vi "Error Tree Value Change and Cycle Numbers.vi"(8 "error in (no error)":errorcluster, 11 "Error Log in":refnum<class "Error Log.lvclass">) -> (0 "error out":errorcluster, 3 "Error Log out":refnum<class "Error Log.lvclass">)   [LabVIEW 2023, in "Data Analysis.lvlib" / "Error Log.lvlib" / "Error Log.lvclass"]
uses:
  Error Log.lvclass
  Error Log.lvclass/Error Log.ctl
  HardwareAbstractionLayer_LVOOP/Database/Database.lvclass
  Data Analysis.lvlib
  <vilib>/Utility/miscctls.llb/LVRowAndColumnUnsignedTypeDef.ctl
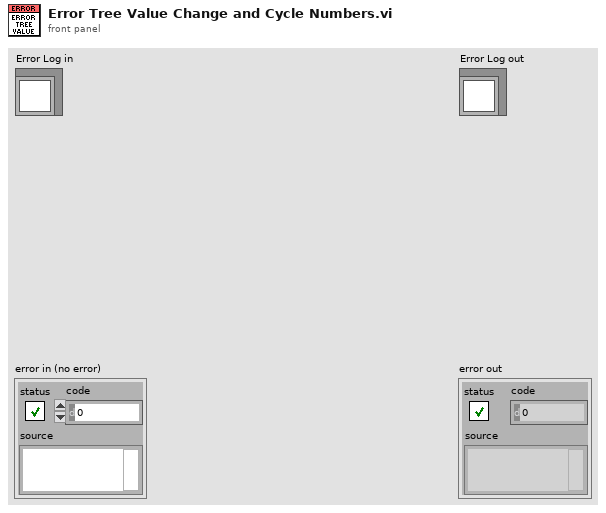
[diagram p1: front panel]
types:
  T1 = typedef "LVRowAndColumnUnsignedTypeDef.ctl" = cluster{"Row":u32, "Column":u32}
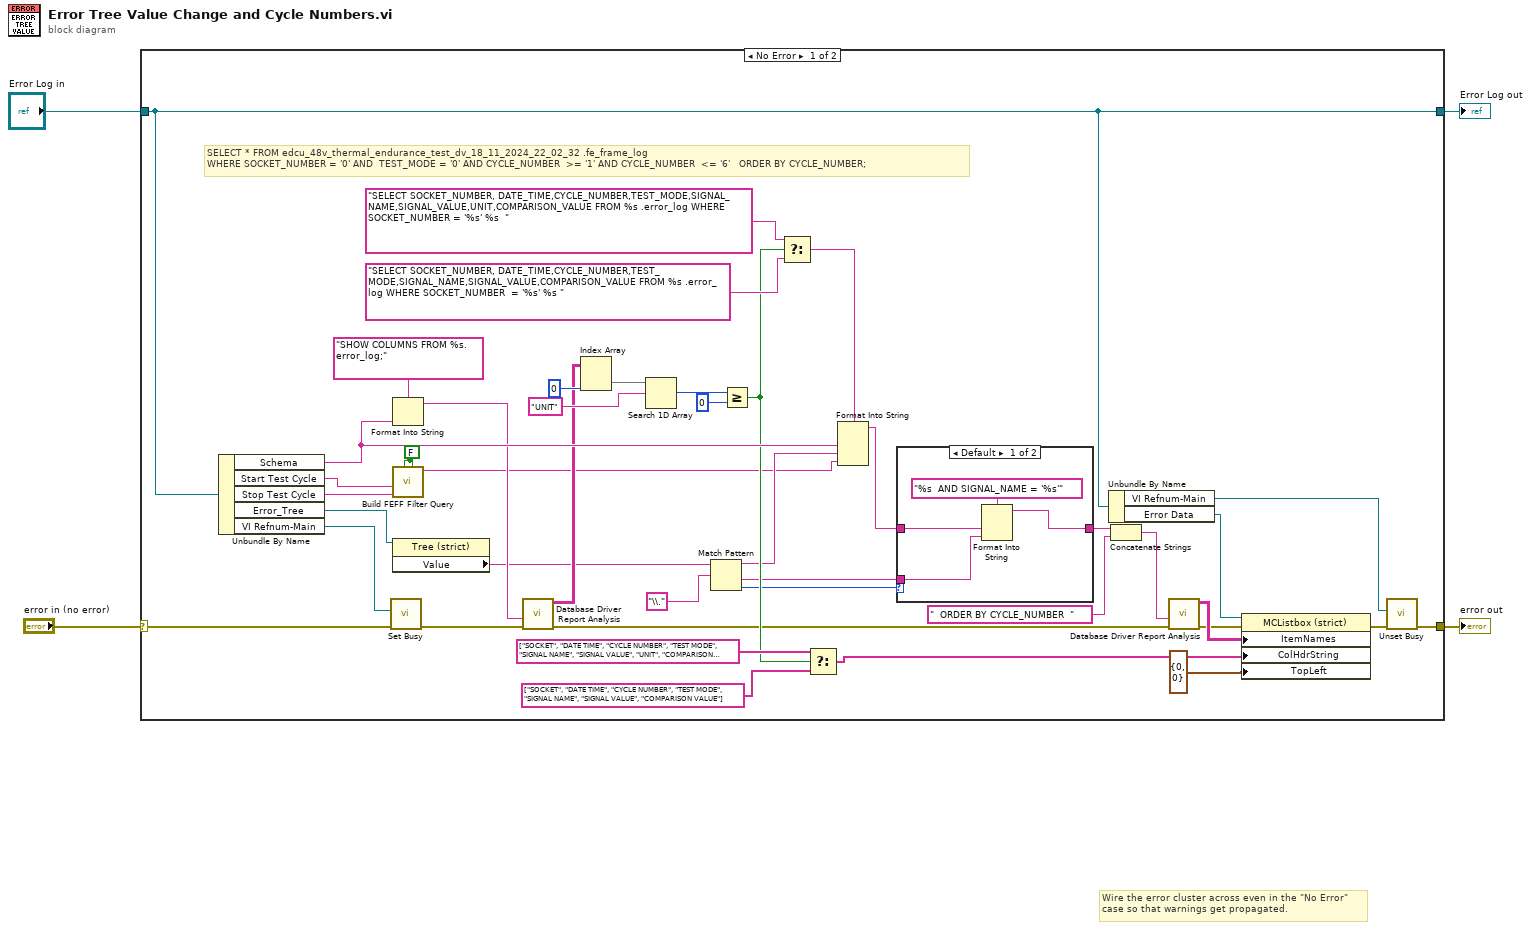
[diagram p0: block diagram]
diagram:
  # "Wire the error cluster across even in the \"No Error\"\ncase so that warnings get propagated."
  n1 = case shown="No Error" "error in (no error)" {
    selector: "error in (no error)" -> [w46 w53]
    tunnel: [w44 w53] -> w3
    tunnel: [w19 w52] -> w1
    tunnel: "Error Log in" -> [w19 w52]
    frame No Error {
      w8 = FALSE ("ORDER BY needed?(Yes)")
      # "SELECT * FROM edcu_48v_thermal_endurance_test_dv_18_11_2024_22_02_32 .fe_frame_log \nWHERE SOCKET_NUMBER = '0' AND  TEST_MODE = '0' AND CYCLE_NUMBER  >= '1' AND CYCLE_NUMBER  <= '6'   ORDER BY CYCLE_NUMBER;"
      n2 = Unbundle By Name(w19) -> ("Schema"=w29:string, "Start Test Cycle"=w42:string, "Stop Test Cycle"=w41:string, "Error_Tree"=w14:refnum<vi>, "VI Refnum-Main"=w40:refnum<vi>)
      n3 = call <vilib>:"Set Busy.vi"("error in (no error)"=w46, "VI reference (current VI)"=w40) -> ("error out"=w23:errorcluster)  [unwired: 8 in, 1 out]
      n4 = Format Into String(format string="SHOW COLUMNS FROM %s.error_log;" ("SQL query"), w29) -> (resulting string=w20:string)  [unwired: 2 in, 1 out]
      n5 = call "Build FEFF Filter Query.vi"("ORDER BY needed?(Yes)"=w8, "WHERE needed?(Yes)"=w8, "Stop Test Cycle"=w41, "Start Test Cycle"=w42) -> ("String"=w6:string)  [unwired: 7 in]
      n6 = property class="Tree (strict)"(reference=w14) -> ("Value"=w13:string)  [unwired: 1 in, 2 out]
      n7 = call "Database Driver Report Analysis.vi"("error in"=w23, "SQL query"=w20) -> ("error out"=w22:errorcluster, "data"=w21:string[][])  [unwired: 6 in, 2 out]
      n8 = Index Array(array=w21, index (col)=0 ("disabled index (col)")) -> (element=w35:string[])  [unwired: 1 in]
      n9 = Search 1D Array(1D array=w35, element="UNIT") -> (index of element=w37:i32)  [unwired: 1 in]
      n10 = Match Pattern(string=w13, regular expression="\\.") -> (before substring=w7:string, after substring=w16:string, offset past match=w17:i32)  [unwired: 1 in, 1 out]
      n11 = Greater Or Equal?(x=w37, y=0) -> (x >= y?=w24:bool)
      n12 = Select(t="SELECT SOCKET_NUMBER, DATE_TIME,CYCLE_NUMBER,TEST_MODE,SIGNAL_NAME,SIGNAL_VALUE,UNIT,COMPARISON_VALUE FROM %s .error_log WHERE SOCKET_NUMBER = '%s' %s  " ("SQL query"), s=w24, f="SELECT SOCKET_NUMBER, DATE_TIME,CYCLE_NUMBER,TEST_MODE,SIGNAL_NAME,SIGNAL_VALUE,COMPARISON_VALUE FROM %s .error_log WHERE SOCKET_NUMBER  = '%s' %s " ("SQL query")) -> (s? t:f=w28:string)
      n13 = Select(t=string[] ["SOCKET", "DATE TIME", "CYCLE NUMBER", "TEST MODE", "SIGNAL NAME", "SIGNAL VALUE", "UNIT", "COMPARISON VALUE"] ("Column Header Strings[]"), s=w24, f=string[] ["SOCKET", "DATE TIME", "CYCLE NUMBER", "TEST MODE", "SIGNAL NAME", "SIGNAL VALUE", "COMPARISON VALUE"] ("Column Header Strings[]")) -> (s? t:f=w26:string[])
      n14 = Format Into String(format string=w28, w29, w7, w6) -> (resulting string=w9:string)  [unwired: 2 in, 1 out]
      n15 = case shown="Default" w17 {
        tunnel: w9 -> [w49 w51]
        tunnel: [w47 w51] -> w12
        tunnel: w16 -> [w48 _]
        frame Default {
          n16 = Format Into String(format string="%s  AND SIGNAL_NAME = '%s'" ("SQL query"), w49, w48) -> (resulting string=w47:string)  [unwired: 2 in, 1 out]
        }
        frame -1 {
        }
      }
      n17 = Unbundle By Name(w19) -> ("VI Refnum-Main"=w43:refnum<vi>, "Error Data"=w15:refnum<vi>)
      n18 = Concatenate Strings(w12, "  ORDER BY CYCLE_NUMBER  ") -> (w11:string)
      n19 = call "Database Driver Report Analysis.vi"("error in"=w22, "SQL query"=w11) -> ("error out"=w38:errorcluster, "data"=w39:string[][])  [unwired: 6 in, 2 out]
      n20 = property class="MCListbox (strict)"(reference=w15, error in=w38, "ItemNames"=w39, "ColHdrString"=w26, "TopLeft"=T1 {"Row"=0, "Column"=0} ("Top Left Visible Cell")) -> (error out=w45:errorcluster)  [unwired: 1 out]
      n21 = call <vilib>:"Unset Busy.vi"("error in (no error)"=w45, "VI reference (current VI)"=w43) -> ("error out"=w44:errorcluster)  [unwired: 9 in]
    }
    frame Error {
    }
  }
  "error out" <- w3
  "Error Log out" <- w1
